vi "Controller_Conditioning_vector.vi"(0 "Angular Offset\n(-180 to 180 or 0 to 360)":dbl, 5 "Min Output(0 to 1)":dbl, 6 "n^x(Unbounded)":dbl=2.5 format="%#_13g", 8 "Enum":T2(ring), 9 "Dead Zone(0 to 1)":dbl, 10 "Y(-1 to 1)":dbl, 11 "X(-1 to 1)":dbl) -> (3 "output cluster":T1)   [LabVIEW 2017]
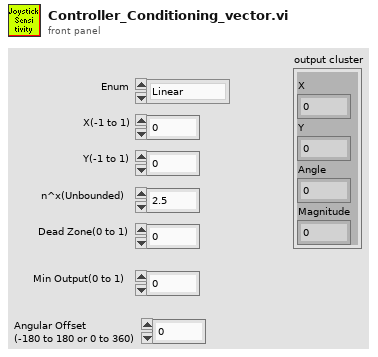
[diagram p1: front panel]
types:
  T1 = cluster{"X":dbl, "Y":dbl, "Angle":dbl, "Magnitude":dbl}
  T2 = enum16{"Linear", "Square  Root", "Square", "n^x"}
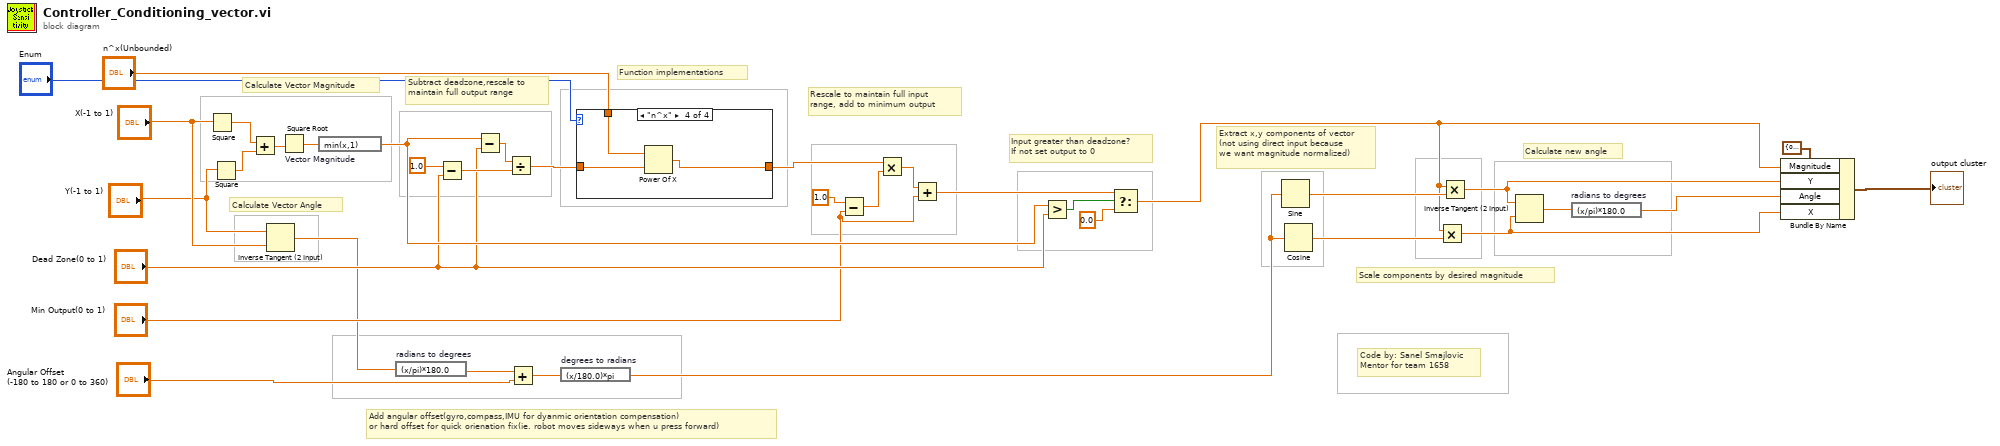
[diagram p0: block diagram]
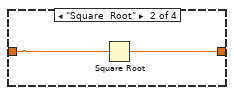
[diagram p3: hidden frame]
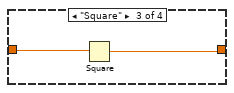
[diagram p4: hidden frame]
diagram:
  # "Add angular offset(gyro,compass,IMU for dyanmic orientation compensation)\nor hard offset for quick orienation fix(ie. robot moves sideways when u press forward)"
  # "Rescale to maintain full input\nrange, add to minimum output"
  # "Subtract deadzone,rescale to \nmaintain full output range"
  # "Code by: Sanel Smajlovic\nMentor for team 1658"
  # "Calculate new angle"
  # "Scale components by desired magnitude"
  # "Extract x,y components of vector\n(not using direct input because\nwe want magnitude normalized)"
  # "Function implementations"
  # "Input greater than deadzone?\nIf not set output to 0"
  # "Calculate Vector Angle"
  # "Calculate Vector Magnitude"
  n1 = Square(x="X(-1 to 1)") -> (x^2=w35:dbl)
  n2 = Square(x="Y(-1 to 1)") -> (x^2=w36:dbl)
  n3 = Add(x=w35, y=w36) -> (x+y=w34:dbl)
  n4 = Inverse Tangent (2 Input)(1:"X(-1 to 1)", 2:"Y(-1 to 1)") -> (0:w5:dbl)
  n5 = Square Root "Vector Magnitude"(x=w34) -> (sqrt(x)=w33:dbl)
  n6 = expression code="min(x,1)"(w33) -> (w23:dbl)
  n7 = expression code="(x/pi)*180.0" "radians to degrees"(w5) -> (w4:dbl)
  n8 = Subtract(x=1.0, y="Dead Zone(0 to 1)") -> (x-y=w19:dbl)
  n9 = Subtract(x=w23, y="Dead Zone(0 to 1)") -> (x-y=w14:dbl)
  n10 = Divide(x=w14, y=w19) -> (x/y=w9:dbl)
  n11 = Add(x=w4, y="Angular Offset\n(-180 to 180 or 0 to 360)") -> (x+y=w2:dbl)
  n12 = expression code="(x/180.0)*pi" "degrees to radians"(w2) -> (w1:dbl)
  n13 = case shown="\"n^x\"" "Enum" {
    tunnel: [w37 w38 w40 w44] -> w8
    tunnel: w9 -> [w37 w39 w41 w43]
    tunnel: "n^x(Unbounded)" -> [_ _ _ w42]
    frame "Linear", Default {
    }
    frame "Square  Root" {
      n14 = Square Root(x=w39) -> (sqrt(x)=w38:dbl)
    }
    frame "Square" {
      n15 = Square(x=w41) -> (x^2=w40:dbl)
    }
    frame "n^x" {
      n16 = Power Of X(1:w43, 2:w42) -> (0:w44:dbl)
    }
  }
  n17 = Subtract(x=1.0, y="Min Output(0 to 1)") -> (x-y=w12:dbl)
  n18 = Multiply(x=w8, y=w12) -> (x*y=w11:dbl)
  n19 = Add(x=w11, y="Min Output(0 to 1)") -> (x+y=w7:dbl)
  n20 = Greater?(x=w23, y="Dead Zone(0 to 1)") -> (0:w25:bool)
  n21 = Select ("Y")(t=w7, s=w25, f=0.0) -> (s? t:f=w6:dbl)
  n22 = Sine(x=w1) -> (sin(x)=w30:dbl)
  n23 = Cosine(x=w1) -> (cos(x)=w29:dbl)
  n24 = Multiply(x=w6, y=w29) -> (x*y=w16:dbl)
  n25 = Multiply(x=w6, y=w30) -> (x*y=w17:dbl)
  n26 = Inverse Tangent (2 Input)(1:w16, 2:w17) -> (0:w26:dbl)
  n27 = expression code="(x/pi)*180.0" "radians to degrees"(w26) -> (w15:dbl)
  n28 = Bundle By Name(cluster=T1 {"X"=0.0, "Y"=0.0, "Angle"=0.0, "Magnitude"=0.0}, "Magnitude"=w6, "Y"=w17, "Angle"=w15, "X"=w16) -> (→"output cluster":T1)
